vi "Design Challenge.vi"() -> ()   [LabVIEW 2025]
panel:
  in  "?":bool
  in  "?":bool
  in  "Launch Angle (Deg)":dbl(knob) min=0.0 max=89.0
  in  "?":bool
  out "XY Graph":cluster{dbl[], dbl[]}[](graph)
  in  "Initial Velocity [m/s]":dbl
  in  "Simba Mass (kg)":dbl
  in  "Pride Rock Height (m)":dbl
  # "ME 235: Design of Microprocessor Based Mechanical Systems"
  # "Lab 2 - Design Challenge (Kyle)"
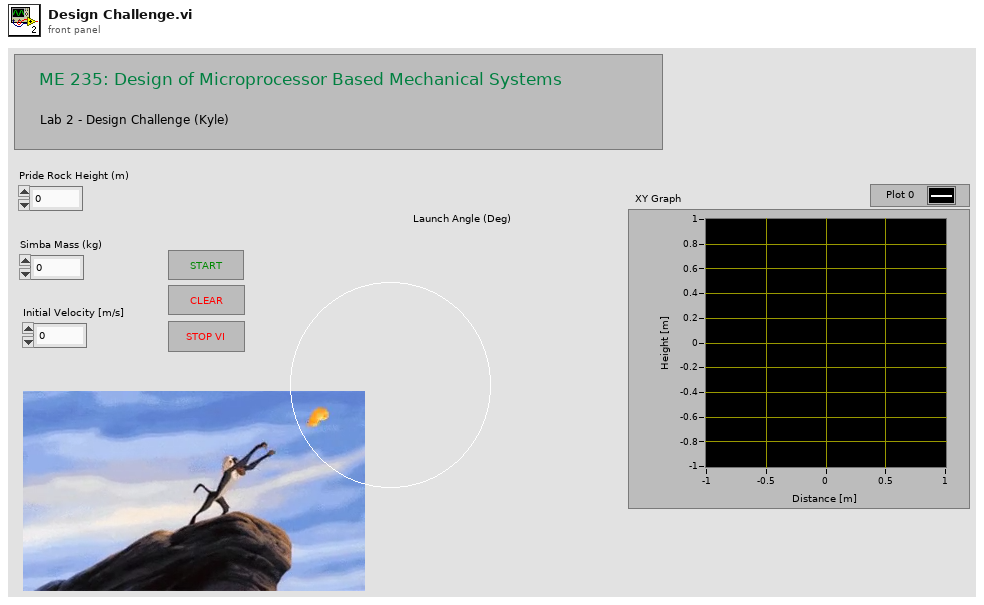
[diagram p1: front panel]
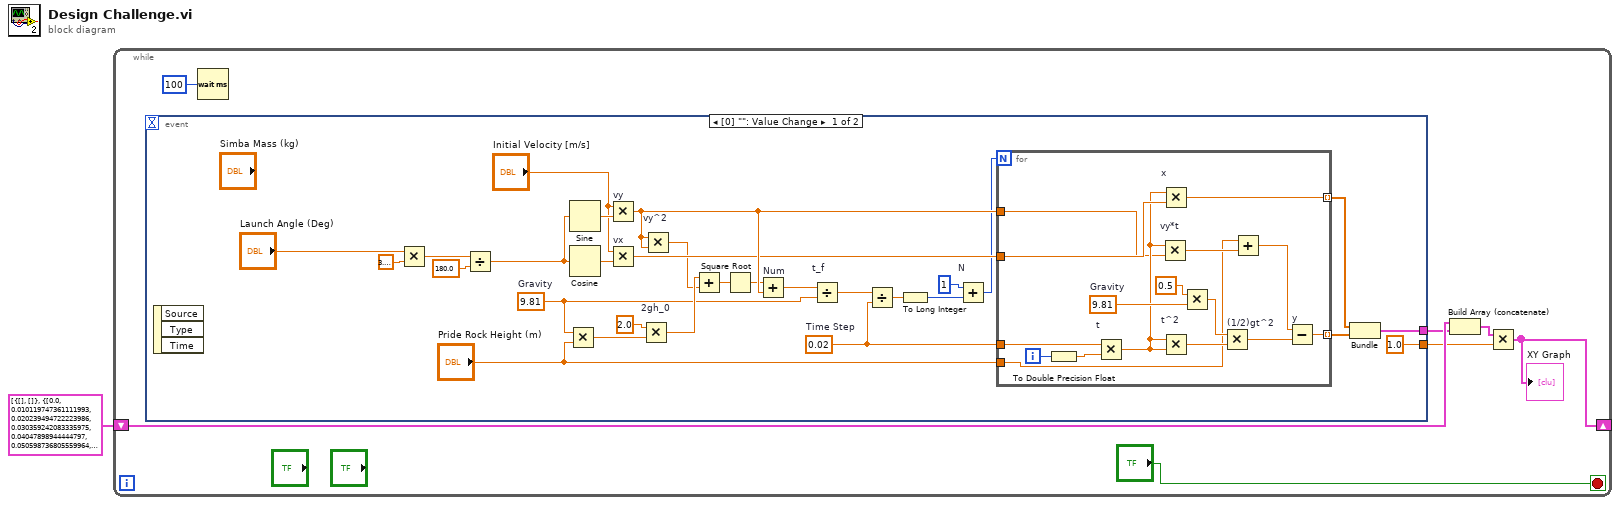
[diagram p0: block diagram]
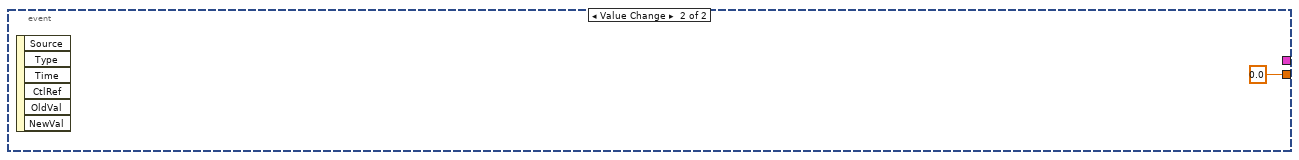
[diagram p2: hidden frame]
diagram:
  n1 = while {
    shift-right: [w3] -> _
    shift-left: cluster{dbl[], dbl[]}[] [{[], []}, {[0.0, 0.010119747361111993, 0.020239494722223986, 0.030359242083335975, 0.04047898944444797, 0.050598736805559964, 0.06071848416667195, 0.07083823152778396, 0.08095797888889594, 0.09107772625000793, 0.10119747361111993, 0.11131722097223191, 0.1214369683333439, 0.1315567156944559, 0.1416764630555679, 0.15179621041667987, 0.16191595777779189, 0.1720357051389039, 0.18215545250001586, 0.19227519986112787, 0.20239494722223986, 0.21251469458335184, 0.22263444194446383, 0.23275418930557584, 0.2428739366666878, 0.2529936840277998, 0.2631134313889118, 0.27323317875002384, 0.2833529261111358, 0.29347267347224776, 0.30359242083335974, 0.3137121681944718, 0.32383191555558377, 0.33395166291669576, 0.3440714102778078, 0.3541911576389198, 0.3643109050000317, 0.3744306523611437, 0.38455039972225574, 0.39467014708336773, 0.4047898944444797, 0.4149096418055917, 0.4250293891667037, 0.43514913652781567, 0.44526888388892766, 0.4553886312500397, 0.4655083786111517, 0.47562812597226367, 0.4857478733333756, 0.49586762069448764, 0.5059873680555996, 0.5161071154167116, 0.5262268627778236, 0.5363466101389356, 0.5464663575000477, 0.5565861048611597, 0.5667058522222717, 0.5768255995833836, 0.5869453469444955, 0.5970650943056075, 0.6071848416667195, 0.6173045890278316, 0.6274243363889436, 0.6375440837500556, 0.6476638311111675, 0.6577835784722795, 0.6679033258333915, 0.6780230731945035, 0.6881428205556156, 0.6982625679167276, 0.7083823152778396, 0.7185020626389514, 0.7286218100000634, 0.7387415573611754, 0.7488613047222874, 0.7589810520833995, 0.7691007994445115, 0.7792205468056235, 0.7893402941667355, 0.7994600415278474, 0.8095797888889594, 0.8196995362500714, 0.8298192836111834, 0.8399390309722955, 0.8500587783334074, 0.8601785256945194, 0.8702982730556313, 0.8804180204167433, 0.8905377677778553], [3.0, 3.137671773541172, 3.2714195470823437, 3.4012433206235158, 3.5271430941646877, 3.6491188677058597, 3.7671706412470316, 3.8812984147882035, 3.9915021883293753, 4.097781961870547, 4.200137735411719, 4.29856950895289, 4.393077282494063, 4.483661056035234, 4.570320829576406, 4.653056603117578, 4.731868376658751, 4.806756150199922, 4.877719923741093, 4.944759697282265, 5.007875470823437, 5.067067244364608, 5.122335017905781, 5.173678791446953, 5.221098564988125, 5.264594338529296, 5.304166112070469, 5.33981388561164, 5.371537659152813, 5.399337432693984, 5.423213206235156, 5.443164979776327, 5.4591927533175, 5.471296526858671, 5.479476300399844, 5.483732073941015, 5.484063847482187, 5.480471621023359, 5.472955394564531, 5.461515168105702, 5.446150941646875, 5.4268627151880455, 5.403650488729218, 5.376514262270391, 5.345454035811562, 5.310469809352734, 5.271561582893906, 5.2287293564350765, 5.1819731299762495, 5.131292903517422, 5.076688677058592, 5.018160450599766, 4.9557082241409365, 4.889331997682109, 4.819031771223281, 4.744807544764451, 4.6666593183056255, 4.584587091846795, 4.498590865387968, 4.408670638929141, 4.314826412470312, 4.217058186011482, 4.115365959552655, 4.009749733093827, 3.900209506634999, 3.786745280176172, 3.6693570537173414, 3.5480448272585132, 3.4228086007996854, 3.293648374340858, 3.160564147882029, 3.0235559214232026, 2.882623694964373, 2.737767468505547, 2.588987242046718, 2.4362830155878896, 2.2796547891290615, 2.119102562670234, 1.9546263362114047, 1.786226109752576, 1.6139018832937477, 1.4376536568349199, 1.2574814303760906, 1.0733852039172636, 0.8853649774584369, 0.6934207509996089, 0.49755252454078125, 0.2977602980819505, 0.09404407162312367]}] ("XY Graph") -> [w7]
    stop <- "?" stop-if-true
    n2 = event shown="[0] \"\": Value Change" {
      selector: _ -> [_ _]
      dyn-events: _ -> [_ _]
      timeout: _ -> [_ _]
      tunnel: [w10 _] -> w6
      tunnel: [1.0 0.0] -> w5
      event Value Change {
        w16 = 0.02  # Time Step
        w14 = 9.81  # Gravity
        n3 = event-data() -> ()  [unwired: 1 in, 3 out]
        n4 = Multiply(x="Launch Angle (Deg)", y=3.141592653589793) -> (x*y=w18:dbl)
        n5 = Divide(x=w18, y=180.0) -> (x/y=w20:dbl)
        n6 = Multiply(x=w14, y="Pride Rock Height (m)") -> (x*y=w23:dbl)
        n7 = Sine(x=w20) -> (sin(x)=w22:dbl)
        n8 = Cosine(x=w20) -> (cos(x)=w19:dbl)
        n9 = Multiply "vy"(x="Initial Velocity [m/s]", y=w22) -> (x*y=w34:dbl)
        n10 = Multiply "vx"(x="Initial Velocity [m/s]", y=w19) -> (x*y=w33:dbl)
        n11 = Multiply "2gh_0"(x=2.0, y=w23) -> (x*y=w25:dbl)
        n12 = Multiply "vy^2"(x=w34, y=w34) -> (x*y=w24:dbl)
        n13 = Add(x=w25, y=w24) -> (x+y=w26:dbl)
        n14 = Square Root(x=w26) -> (sqrt(x)=w27:dbl)
        n15 = Add "Num"(x=w27, y=w34) -> (x+y=w28:dbl)
        n16 = Divide "t_f"(x=w28, y=w14) -> (x/y=w29:dbl)
        n17 = Divide(x=w29, y=w16) -> (x/y=w30:dbl)
        n18 = To Long Integer(number=w30) -> (32bit integer=w31:i32)
        n19 = Add "N"(x=1, y=w31) -> (x+y=w32:i32)
        n20 = for {
          N: w32 -> [_]
          tunnel: w16 -> [w53]
          tunnel: w33 -> [w50]
          tunnel: w34 -> [w44]
          tunnel: [w40] -> w37 mode=indexing
          tunnel: [w39] -> w36 mode=indexing
          tunnel: "Pride Rock Height (m)" -> [w38]
          i -> [w51]
          w48 = 9.81  # Gravity
          n21 = To Double Precision Float(number=w51) -> (double precision float=w52:dbl)
          n22 = Multiply "t"(x=w53, y=w52) -> (x*y=w45:dbl)
          n23 = Multiply "vy*t"(x=w45, y=w44) -> (x*y=w43:dbl)
          n24 = Multiply "x"(x=w45, y=w50) -> (x*y=w40:dbl)
          n25 = Multiply "t^2"(x=w45, y=w45) -> (x*y=w46:dbl)
          n26 = Multiply(x=0.5, y=w48) -> (x*y=w47:dbl)
          n27 = Multiply "(1/2)gt^2"(x=w47, y=w46) -> (x*y=w42:dbl)
          n28 = Add(x=w38, y=w43) -> (x+y=w41:dbl)
          n29 = Subtract "y"(x=w41, y=w42) -> (x-y=w39:dbl)
        }
        n30 = Bundle(w37, w36) -> (w10:cluster{dbl[], dbl[]})  [unwired: 1 in]
      }
      event Value Change {
        n31 = event-data() -> ()  [unwired: 1 in, 6 out]
      }
    }
    n32 = Wait (ms)(milliseconds to wait=u32 100) -> ()  [unwired: 1 out]
    n33 = Build Array (concatenate)(w7, w6) -> (w4:cluster{dbl[], dbl[]}[])
    n34 = Multiply(x=w4, y=w5) -> (x*y=w3:cluster{dbl[], dbl[]}[])
    "XY Graph" <- w3
  }
